vi "Apply Theme.vi"(8 "Error In":errorcluster, 10 "Override Root With (Empty)":string, 11 "Appearance Actor in":refnum<class "Appearance Actor.lvclass">) -> (0 "Error Out":errorcluster, 3 "Appearance Actor out":refnum<class "Appearance Actor.lvclass">)   [LabVIEW 2021, in "Appearance Actor.lvlib" / "Appearance Actor.lvclass"]
doc: "Apply the loaded theme to the current Actor.\n\nBy default, needs UI Control References to be listed in <B>Appearance Actor</B> internal data. But you can override this vi to do it your own way."
uses:
  Appearance Actor.lvclass
  Appearance Actor.lvclass/Appearance Actor.ctl
  Theme Classes/Generic Theme/Generic Theme.lvclass
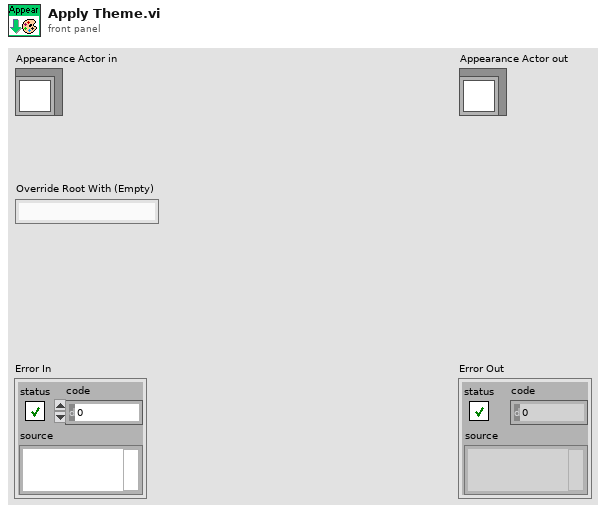
[diagram p1: front panel]
types:
  T1 = typedef "Appearance Actor.lvlib/Appearance Actor.lvclass/UI Controls--map.ctl" = map{string, T2}
  T2 = typedef "Appearance Actor.lvlib/Appearance Actor.lvclass/Element Controls--map.ctl" = map{string, T3}
  T3 = typedef "Appearance Actor.lvlib/Appearance Actor.lvclass/Controls--map.ctl" = map{string, refnum<vi>}
  T4 = typedef "Appearance Actor.lvlib/Appearance Actor.lvclass/UI Panes--map.ctl" = map{string, T5}
  T5 = typedef "Appearance Actor.lvlib/Appearance Actor.lvclass/Element Panes--map.ctl" = map{string, T6}
  T6 = typedef "Appearance Actor.lvlib/Appearance Actor.lvclass/Panes--map.ctl" = map{string, refnum<vi>}
  T7 = typedef "Appearance Actor.lvlib/Appearance Actor.lvclass/UI Splitters--map.ctl" = map{string, T8}
  T8 = typedef "Appearance Actor.lvlib/Appearance Actor.lvclass/Element Splitters--map.ctl" = map{string, T9}
  T9 = typedef "Appearance Actor.lvlib/Appearance Actor.lvclass/Splitters--map.ctl" = map{string, refnum<vi>}
  T10 = typedef "Appearance Actor.lvlib/Generic Theme.lvclass/Window Element--enum.ctl" = enum16{"None", "TB", "SM", "BP", "SB"}
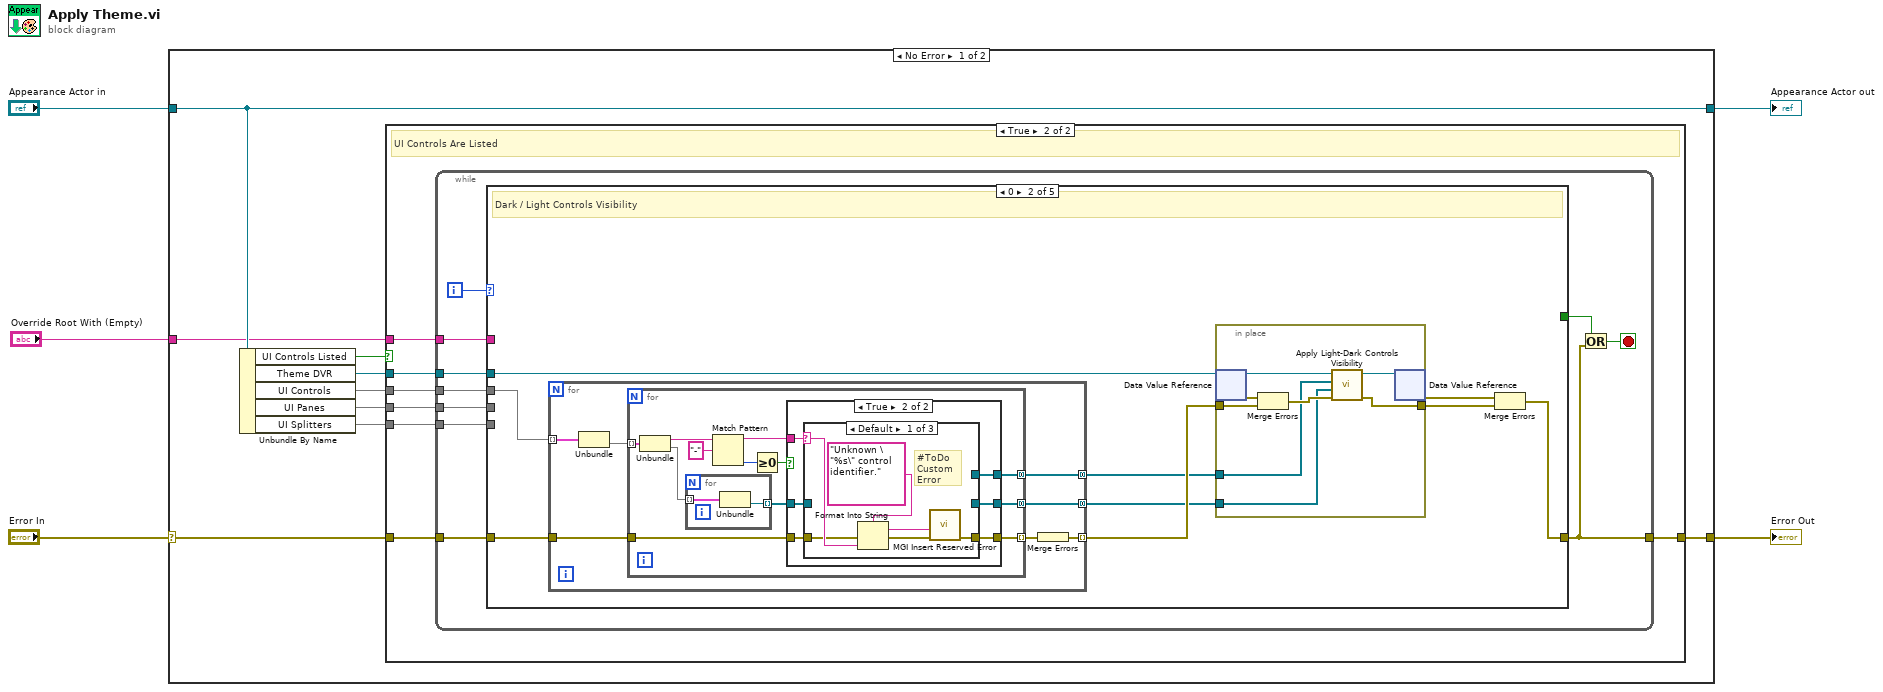
[diagram p0: block diagram]
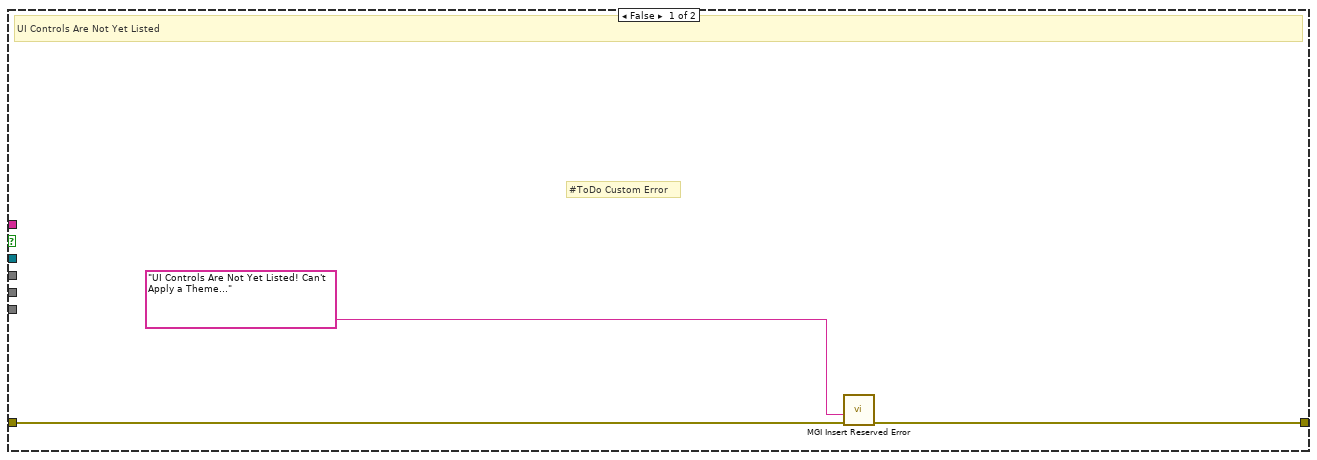
[diagram p2: hidden frame]
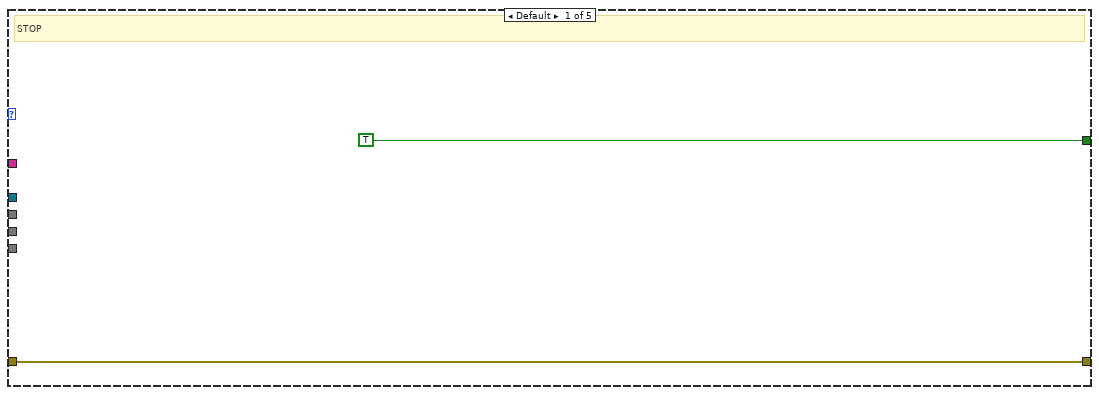
[diagram p3: hidden frame]
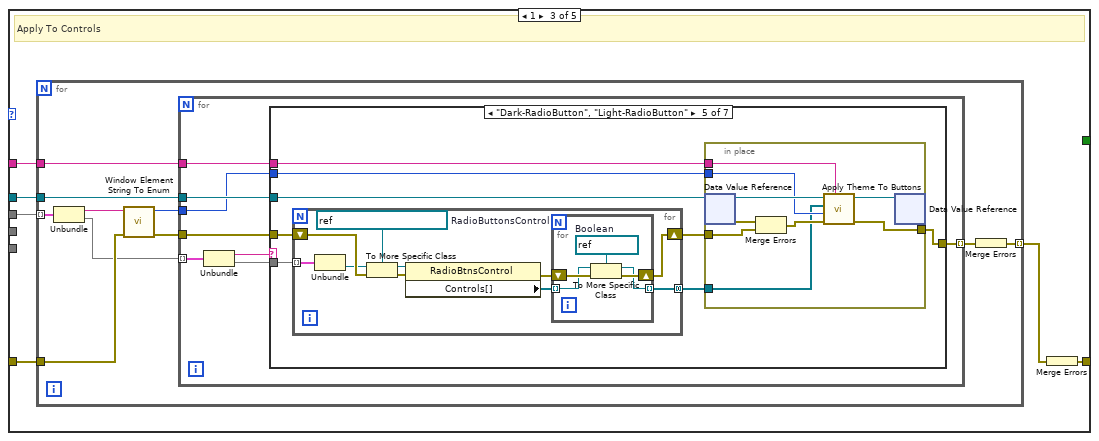
[diagram p7: hidden frame]
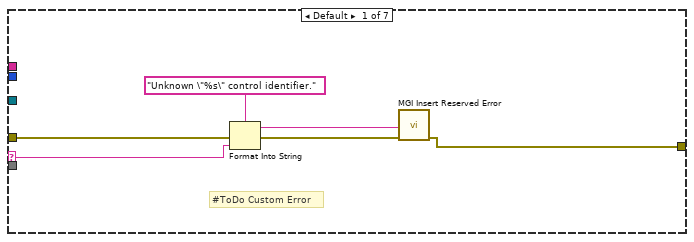
[diagram p8: hidden frame]
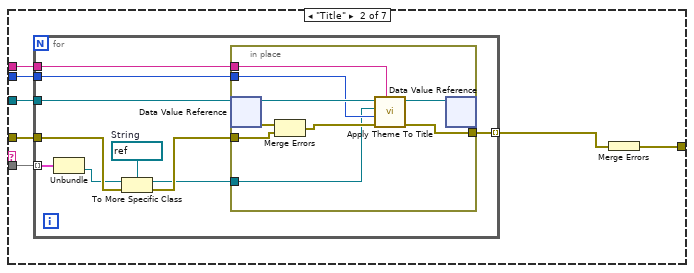
[diagram p9: hidden frame]
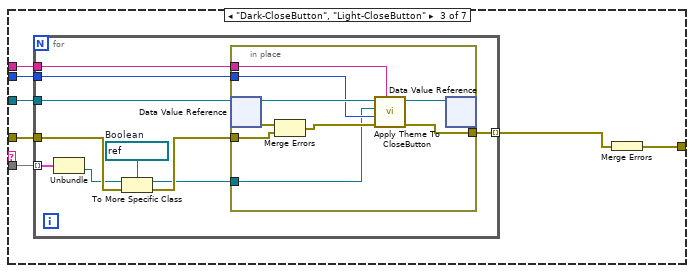
[diagram p10: hidden frame]
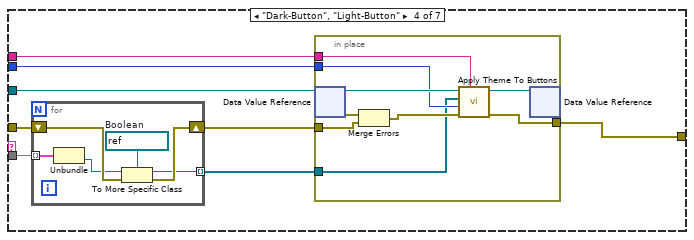
[diagram p11: hidden frame]
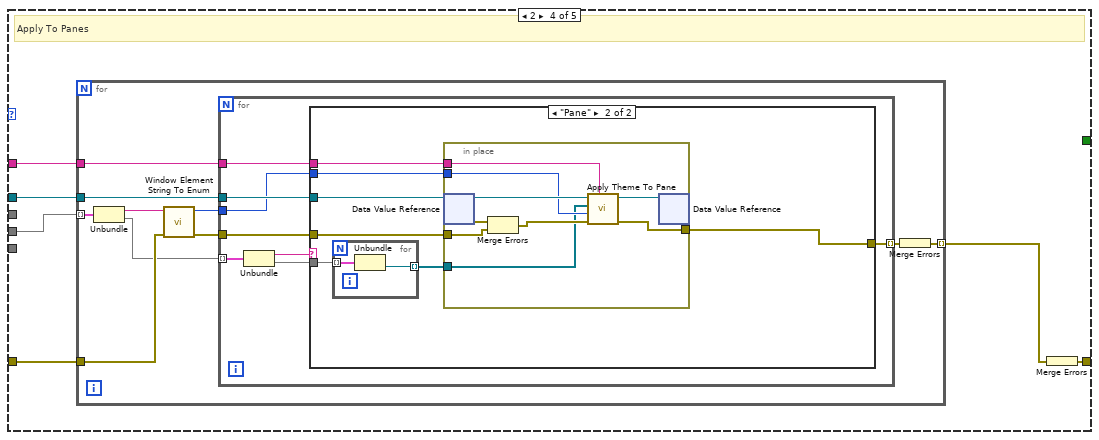
[diagram p14: hidden frame]
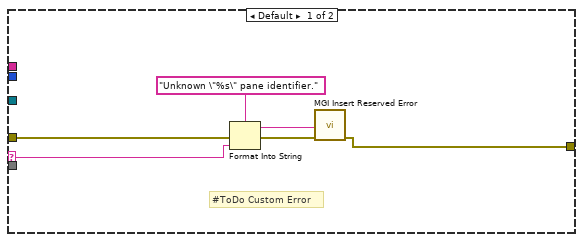
[diagram p15: hidden frame]
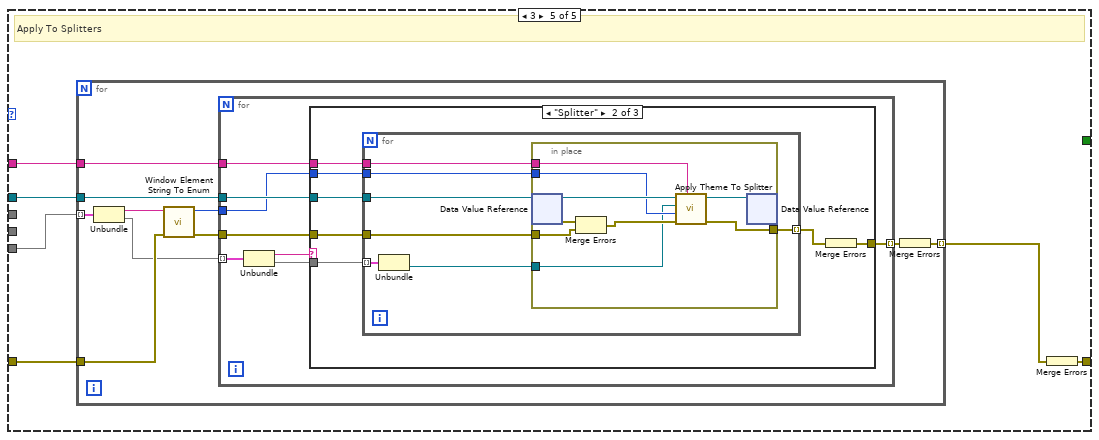
[diagram p16: hidden frame]
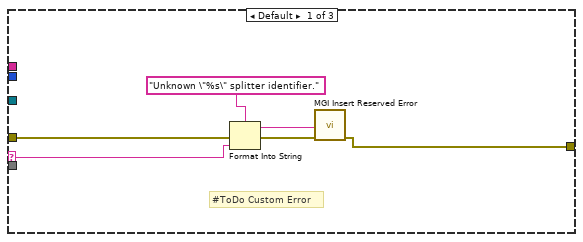
[diagram p17: hidden frame]
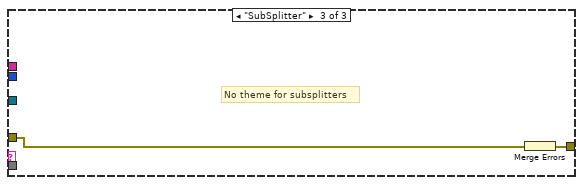
[diagram p18: hidden frame]
diagram:
  n1 = case shown="No Error" "Error In" {
    selector: "Error In" -> [w12 w335]
    tunnel: [w11 w335] -> w4
    tunnel: [w14 w334] -> w2
    tunnel: "Appearance Actor in" -> [w14 w334]
    tunnel: "Override Root With (Empty)" -> [w9 _]
    frame No Error {
      n2 = Unbundle By Name(w14) -> ("UI Controls Listed"=w10:bool, "Theme DVR"=w13:refnum<data-value>, "UI Controls"=w8:T1, "UI Panes"=w7:T4, "UI Splitters"=w6:T7)
      n3 = case shown="True" w10 {
        tunnel: w13 -> [_ w23]
        tunnel: w12 -> [w17 w21]
        tunnel: [w16 w24] -> w11
        tunnel: w9 -> [_ w22]
        tunnel: w8 -> [_ w20]
        tunnel: w7 -> [_ w19]
        tunnel: w6 -> [_ w18]
        frame False {
          # "#ToDo Custom Error"
          # "UI Controls Are Not Yet Listed"
          n4 = call <userlib>:"MGI Insert Reserved Error.vi"("Error In"=w17, "Error Description"="UI Controls Are Not Yet Listed! Can't Apply a Theme..." ("format string")) -> ("Error Out"=w16:errorcluster)  [unwired: 9 in]
        }
        frame True {
          # "UI Controls Are Listed"
          n5 = while {
            tunnel: w23 -> [w33]
            tunnel: w21 -> [w29]
            tunnel: [w30] -> w24
            tunnel: w22 -> [w28]
            tunnel: w20 -> [w27]
            tunnel: w19 -> [w26]
            tunnel: w18 -> [w25]
            i -> [w34]
            stop <- w31 stop-if-true
            n6 = case shown="0" w34 {
              tunnel: w33 -> [_ w42 w97 w236 w284]
              tunnel: [TRUE _ _ _ _] -> w32
              tunnel: w29 -> [w35 w40 w94 w234 w282]
              tunnel: [w35 w43 w92 w232 w280] -> w30
              tunnel: w28 -> [_ _ w95 w235 w283]
              tunnel: w27 -> [_ w41 w96 _ _]
              tunnel: w26 -> [_ _ _ w231 _]
              tunnel: w25 -> [_ _ _ _ w279]
              frame Default {
                # "STOP"
              }
              frame 0 {
                # "Dark / Light Controls Visibility"
                n7 = for {
                  tunnel: w41 -> [w52] mode=indexing
                  tunnel: w40 -> [w50]
                  tunnel: [w48] -> w39 mode=indexing
                  tunnel: [w47] -> w38 mode=concatenating
                  tunnel: [w46] -> w37 mode=concatenating
                  n8 = Unbundle(w52) -> ("Element Controls"=w51:T2)  [unwired: 1 out]
                  n9 = for {
                    tunnel: w51 -> [w64] mode=indexing
                    tunnel: w50 -> [w60]
                    tunnel: [w57] -> w49 mode=indexing
                    tunnel: [w54] -> w47 mode=concatenating
                    tunnel: [w53] -> w46 mode=concatenating
                    n10 = Unbundle(w64) -> ("Key"=w63:string, "Controls"=w56:T3)
                    n11 = for {
                      tunnel: w56 -> [w66] mode=indexing
                      tunnel: [w65] -> w55 mode=indexing
                      n12 = Unbundle(w66) -> ("Ctl Refnum"=w65:refnum<vi>)  [unwired: 1 out]
                    }
                    n13 = Match Pattern(string=w63, regular expression="-") -> (before substring=w58:string, offset past match=w61:i32)  [unwired: 1 in, 2 out]
                    n14 = Greater Or Equal To 0?(x=w61) -> (x >= 0?=w59:bool)
                    n15 = case shown="True" w59 {
                      tunnel: w60 -> [w67 w73]
                      tunnel: w58 -> [_ w71]
                      tunnel: [w67 w72] -> w57
                      tunnel: w55 -> [_ w70]
                      tunnel: [_ w69] -> w54
                      tunnel: [_ w68] -> w53
                      frame False {
                      }
                      frame True {
                        n16 = case shown="Default" w71 {
                          selector: w71 -> [w76 _ _]
                          tunnel: [w79 w81 w82] -> w72
                          tunnel: w73 -> [w75 w81 w82]
                          tunnel: w70 -> [_ w80 w83]
                          tunnel: [_ _ w83] -> w69
                          tunnel: [_ w80 _] -> w68
                          frame Default {
                            # "#ToDo Custom Error"
                            n17 = Format Into String(format string="Unknown \"%s\" control identifier.", error in=w75, w76) -> (resulting string=w77:string, error out=w74:errorcluster)  [unwired: 1 in]
                            n18 = call <userlib>:"MGI Insert Reserved Error.vi"("Error In"=w74, "Error Description"=w77) -> ("Error Out"=w79:errorcluster)  [unwired: 9 in]
                          }
                          frame "Light" {
                          }
                          frame "Dark" {
                          }
                        }
                      }
                    }
                  }
                  n19 = Merge Errors(w49) -> (w48:errorcluster)
                }
                n20 = in-place {
                  in-place-border: [w90] -> w44
                  in-place-border: w39 -> [w86]
                  in-place-border: w38 -> [w85]
                  in-place-border: w37 -> [w84]
                  n21 = in-place-dvr #1(w42) -> (w89:refnum<class "Generic Theme.lvclass">, w88:errorcluster)
                  n22 = Merge Errors(w88, w86) -> (w87:errorcluster)
                  n23 = call-dynamic "Apply Light-Dark Controls Visibility.vi"("Error In"=w87, "Dark Controls"=w85, "Light Controls"=w84, "Generic Theme in"=w89) -> ("Error Out"=w90:errorcluster, "Generic Theme out"=w91:refnum<class "Generic Theme.lvclass">)  [unwired: 6 in]
                  n24 = in-place-dvr #1(w91) -> (w45:errorcluster)  [unwired: 1 out]
                }
                n25 = Merge Errors(w45, w44) -> (w43:errorcluster)
              }
              frame 1 {
                # "Apply To Controls"
                n26 = for {
                  tunnel: w97 -> [w106]
                  tunnel: w96 -> [w105] mode=indexing
                  tunnel: w95 -> [w103]
                  tunnel: w94 -> [w107]
                  tunnel: [w98] -> w93 mode=indexing
                  n27 = Unbundle(w105) -> ("Key"=w102:string, "Element Controls"=w104:T2)
                  n28 = call "Window Element String To Enum.vi"("Error In"=w107, "Window Element Str"=w102) -> ("Error Out"=w100:errorcluster, "Window Element"=w101:T10)  [unwired: 8 in]
                  n29 = for {
                    tunnel: w106 -> [w115]
                    tunnel: w104 -> [w114] mode=indexing
                    tunnel: w103 -> [w113]
                    tunnel: w101 -> [w112]
                    tunnel: w100 -> [w111]
                    tunnel: [w108] -> w99 mode=indexing
                    n30 = Unbundle(w114) -> ("Key"=w110:string, "Controls"=w109:T3)
                    n31 = case shown="\"Dark-RadioButton\", \"Light-RadioButton\"" w110 {
                      selector: w110 -> [w118 _ _ _ _ _ _]
                      tunnel: w115 -> [_ w128 w154 w181 w204 _ _]
                      tunnel: w113 -> [_ w127 w153 w180 w203 _ _]
                      tunnel: w112 -> [_ w126 w152 w179 w202 _ _]
                      tunnel: w111 -> [w121 w125 w151 w178 w201 w229 w230]
                      tunnel: w109 -> [_ w124 w150 w177 w200 _ _]
                      tunnel: [w116 w122 w148 w174 w197 w229 w230] -> w108
                      frame Default {
                        # "#ToDo Custom Error"
                        n32 = Format Into String(format string="Unknown \"%s\" control identifier.", error in=w121, w118) -> (resulting string=w119:string, error out=w120:errorcluster)  [unwired: 1 in]
                        n33 = call <userlib>:"MGI Insert Reserved Error.vi"("Error In"=w120, "Error Description"=w119) -> ("Error Out"=w116:errorcluster)  [unwired: 9 in]
                      }
                      frame "Title" {
                        n34 = for {
                          tunnel: w128 -> [w138]
                          tunnel: w127 -> [w137]
                          tunnel: w126 -> [w136]
                          tunnel: w125 -> [w135]
                          tunnel: w124 -> [w131] mode=indexing
                          tunnel: [w129] -> w123 mode=indexing
                          w133 = refnum<vi> refnum  # String
                          n35 = Unbundle(w131) -> ("Ctl Refnum"=w130:refnum<vi>)  [unwired: 1 out]
                          n36 = To More Specific Class(target class=w133, reference=w130, error in=w135) -> (specific class reference=w132:refnum<vi>, error out=w134:errorcluster)
                          n37 = in-place {
                            in-place-border: [w144] -> w129
                            in-place-border: w137 -> [w143]
                            in-place-border: w136 -> [w142]
                            in-place-border: w134 -> [w140]
                            in-place-border: w132 -> [w139]
                            n38 = in-place-dvr #2(w138) -> (w147:refnum<class "Generic Theme.lvclass">, w146:errorcluster)
                            n39 = Merge Errors(w146, w140) -> (w141:errorcluster)
                            n40 = call-dynamic "Apply Theme To Title.vi"("Override Root With (Empty)"=w143, "Error In"=w141, "Window Element"=w142, "Title Ref"=w139, "Generic Theme in"=w147) -> ("Error Out"=w144:errorcluster, "Generic Theme out"=w145:refnum<class "Generic Theme.lvclass">)  [unwired: 5 in]
                            n41 = in-place-dvr #2(w145) -> ()  [unwired: 2 out]
                          }
                        }
                        n42 = Merge Errors(w123) -> (w122:errorcluster)
                      }
                      frame "Dark-CloseButton", "Light-CloseButton" {
                        n43 = for {
                          tunnel: w154 -> [w164]
                          tunnel: w153 -> [w163]
                          tunnel: w152 -> [w162]
                          tunnel: w151 -> [w161]
                          tunnel: w150 -> [w157] mode=indexing
                          tunnel: [w155] -> w149 mode=indexing
                          w159 = refnum<vi> refnum  # Boolean
                          n44 = Unbundle(w157) -> ("Ctl Refnum"=w156:refnum<vi>)  [unwired: 1 out]
                          n45 = To More Specific Class(target class=w159, reference=w156, error in=w161) -> (specific class reference=w158:refnum<vi>, error out=w160:errorcluster)
                          n46 = in-place {
                            in-place-border: [w170] -> w155
                            in-place-border: w163 -> [w169]
                            in-place-border: w162 -> [w168]
                            in-place-border: w160 -> [w166]
                            in-place-border: w158 -> [w165]
                            n47 = in-place-dvr #3(w164) -> (w173:refnum<class "Generic Theme.lvclass">, w172:errorcluster)
                            n48 = Merge Errors(w172, w166) -> (w167:errorcluster)
                            n49 = call-dynamic "Apply Theme To CloseButton.vi"("Override Root With (Empty)"=w169, "Error In"=w167, "Window Element"=w168, "CloseButton Ref"=w165, "Generic Theme in"=w173) -> ("Error Out"=w170:errorcluster, "Generic Theme out"=w171:refnum<class "Generic Theme.lvclass">)  [unwired: 5 in]
                            n50 = in-place-dvr #3(w171) -> ()  [unwired: 2 out]
                          }
                        }
                        n51 = Merge Errors(w149) -> (w148:errorcluster)
                      }
                      frame "Dark-Button", "Light-Button" {
                        n52 = for {
                          tunnel: w177 -> [w186] mode=indexing
                          tunnel: [w183] -> w175 mode=indexing
                          shift-right: [w185] -> w176
                          shift-left: w178 -> [w187]
                          w184 = refnum<vi> refnum  # Boolean
                          n53 = Unbundle(w186) -> ("Ctl Refnum"=w182:refnum<vi>)  [unwired: 1 out]
                          n54 = To More Specific Class(target class=w184, reference=w182, error in=w187) -> (specific class reference=w183:refnum<vi>, error out=w185:errorcluster)
                        }
                        n55 = in-place {
                          in-place-border: [w193] -> w174
                          in-place-border: w180 -> [w192]
                          in-place-border: w179 -> [w191]
                          in-place-border: w176 -> [w189]
                          in-place-border: w175 -> [w188]
                          n56 = in-place-dvr #4(w181) -> (w196:refnum<class "Generic Theme.lvclass">, w195:errorcluster)
                          n57 = Merge Errors(w195, w189) -> (w190:errorcluster)
                          n58 = call-dynamic "Apply Theme To Buttons.vi"("Override Root With (Empty)"=w192, "Error In"=w190, "Window Element"=w191, "Buttons Ref"=w188, "Generic Theme in"=w196) -> ("Error Out"=w193:errorcluster, "Generic Theme out"=w194:refnum<class "Generic Theme.lvclass">)  [unwired: 5 in]
                          n59 = in-place-dvr #4(w194) -> ()  [unwired: 2 out]
                        }
                      }
                      frame "Dark-RadioButton", "Light-RadioButton" {
                        n60 = for {
                          tunnel: w200 -> [w213] mode=indexing
                          tunnel: [w205] -> w198 mode=concatenating
                          shift-right: [w206] -> w199
                          shift-left: w201 -> [w214]
                          w212 = refnum<vi> refnum  # RadioButtonsControl
                          n61 = Unbundle(w213) -> ("Ctl Refnum"=w211:refnum<vi>)  [unwired: 1 out]
                          n62 = To More Specific Class(target class=w212, reference=w211, error in=w214) -> (specific class reference=w210:refnum<vi>, error out=w209:errorcluster)
                          n63 = property class="RadioBtnsControl"(reference=w210, error in=w209) -> (error out=w207:errorcluster, "Controls[]"=w208:refnum<vi>[])  [unwired: 1 out]
                          n64 = for {
                            tunnel: w208 -> [w217] mode=indexing
                            shift-right: [w218] -> w206
                            shift-left: w207 -> [w219]
                            tunnel: [w216] -> w205 mode=indexing
                            w215 = refnum<vi> refnum  # Boolean
                            n65 = To More Specific Class(target class=w215, reference=w217, error in=w219) -> (specific class reference=w216:refnum<vi>, error out=w218:errorcluster)
                          }
                        }
                        n66 = in-place {
                          in-place-border: [w225] -> w197
                          in-place-border: w203 -> [w224]
                          in-place-border: w202 -> [w223]
                          in-place-border: w199 -> [w221]
                          in-place-border: w198 -> [w220]
                          n67 = in-place-dvr #5(w204) -> (w228:refnum<class "Generic Theme.lvclass">, w227:errorcluster)
                          n68 = Merge Errors(w227, w221) -> (w222:errorcluster)
                          n69 = call-dynamic "Apply Theme To Buttons.vi"("Override Root With (Empty)"=w224, "Error In"=w222, "Window Element"=w223, "Buttons Ref"=w220, "Generic Theme in"=w228) -> ("Error Out"=w225:errorcluster, "Generic Theme out"=w226:refnum<class "Generic Theme.lvclass">)  [unwired: 5 in]
                          n70 = in-place-dvr #5(w226) -> ()  [unwired: 2 out]
                        }
                      }
                      frame "SubPanel" {
                        # "No theme for SubPanels"
                      }
                      frame "Icon" {
                        # "No theme for Icon"
                      }
                    }
                  }
                  n71 = Merge Errors(w99) -> (w98:errorcluster)
                }
                n72 = Merge Errors(w93) -> (w92:errorcluster)
              }
              frame 2 {
                # "Apply To Panes"
                n73 = for {
                  tunnel: w236 -> [w245]
                  tunnel: w231 -> [w244] mode=indexing
                  tunnel: w235 -> [w242]
                  tunnel: w234 -> [w246]
                  tunnel: [w237] -> w233 mode=indexing
                  n74 = Unbundle(w244) -> ("Key"=w241:string, "Element Panes"=w243:T5)
                  n75 = call "Window Element String To Enum.vi"("Error In"=w246, "Window Element Str"=w241) -> ("Error Out"=w239:errorcluster, "Window Element"=w240:T10)  [unwired: 8 in]
                  n76 = for {
                    tunnel: w245 -> [w254]
                    tunnel: w243 -> [w253] mode=indexing
                    tunnel: w242 -> [w252]
                    tunnel: w240 -> [w251]
                    tunnel: w239 -> [w250]
                    tunnel: [w247] -> w238 mode=indexing
                    n77 = Unbundle(w253) -> ("Key"=w249:string, "Panes"=w248:T6)
                    n78 = case shown="\"Pane\"" w249 {
                      selector: w249 -> [w257 _]
                      tunnel: w254 -> [_ w267]
                      tunnel: w252 -> [_ w266]
                      tunnel: w251 -> [_ w265]
                      tunnel: w250 -> [w260 w261]
                      tunnel: w248 -> [_ w264]
                      tunnel: [w255 w262] -> w247
                      frame Default {
                        # "#ToDo Custom Error"
                        n79 = Format Into String(format string="Unknown \"%s\" pane identifier.", error in=w260, w257) -> (resulting string=w258:string, error out=w259:errorcluster)  [unwired: 1 in]
                        n80 = call <userlib>:"MGI Insert Reserved Error.vi"("Error In"=w259, "Error Description"=w258) -> ("Error Out"=w255:errorcluster)  [unwired: 9 in]
                      }
                      frame "Pane" {
                        n81 = for {
                          tunnel: w264 -> [w269] mode=indexing
                          tunnel: [w268] -> w263 mode=indexing
                          n82 = Unbundle(w269) -> ("Pane Refnum"=w268:refnum<vi>)  [unwired: 1 out]
                        }
                        n83 = in-place {
                          in-place-border: [w275] -> w262
                          in-place-border: w266 -> [w274]
                          in-place-border: w265 -> [w273]
                          in-place-border: w261 -> [w271]
                          in-place-border: w263 -> [w270]
                          n84 = in-place-dvr #6(w267) -> (w278:refnum<class "Generic Theme.lvclass">, w277:errorcluster)
                          n85 = Merge Errors(w277, w271) -> (w272:errorcluster)
                          n86 = call-dynamic "Apply Theme To Pane.vi"("Override Root With (Empty)"=w274, "Error In"=w272, "Window Element"=w273, "Pane Refs"=w270, "Generic Theme in"=w278) -> ("Error Out"=w275:errorcluster, "Generic Theme out"=w276:refnum<class "Generic Theme.lvclass">)  [unwired: 5 in]
                          n87 = in-place-dvr #6(w276) -> ()  [unwired: 2 out]
                        }
                      }
                    }
                  }
                  n88 = Merge Errors(w238) -> (w237:errorcluster)
                }
                n89 = Merge Errors(w233) -> (w232:errorcluster)
              }
              frame 3 {
                # "Apply To Splitters"
                n90 = for {
                  tunnel: w284 -> [w293]
                  tunnel: w279 -> [w292] mode=indexing
                  tunnel: w283 -> [w290]
                  tunnel: w282 -> [w294]
                  tunnel: [w285] -> w281 mode=indexing
                  n91 = Unbundle(w292) -> ("Key"=w289:string, "Element Splitters"=w291:T8)
                  n92 = call "Window Element String To Enum.vi"("Error In"=w294, "Window Element Str"=w289) -> ("Error Out"=w287:errorcluster, "Window Element"=w288:T10)  [unwired: 8 in]
                  n93 = for {
                    tunnel: w293 -> [w302]
                    tunnel: w291 -> [w301] mode=indexing
                    tunnel: w290 -> [w300]
                    tunnel: w288 -> [w299]
                    tunnel: w287 -> [w298]
                    tunnel: [w295] -> w286 mode=indexing
                    n94 = Unbundle(w301) -> ("Key"=w297:string, "Splitters"=w296:T9)
                    n95 = case shown="\"Splitter\"" w297 {
                      selector: w297 -> [w305 _ _]
                      tunnel: w302 -> [_ w315 _]
                      tunnel: w300 -> [_ w314 _]
                      tunnel: w299 -> [_ w313 _]
                      tunnel: w298 -> [w308 w312 w332]
                      tunnel: w296 -> [_ w311 _]
                      tunnel: [w303 w309 w333] -> w295
                      frame Default {
                        # "#ToDo Custom Error"
                        n96 = Format Into String(format string="Unknown \"%s\" splitter identifier.", error in=w308, w305) -> (resulting string=w306:string, error out=w307:errorcluster)  [unwired: 1 in]
                        n97 = call <userlib>:"MGI Insert Reserved Error.vi"("Error In"=w307, "Error Description"=w306) -> ("Error Out"=w303:errorcluster)  [unwired: 9 in]
                      }
                      frame "Splitter" {
                        n98 = for {
                          tunnel: w315 -> [w322]
                          tunnel: w314 -> [w321]
                          tunnel: w313 -> [w320]
                          tunnel: w312 -> [w319]
                          tunnel: w311 -> [w318] mode=indexing
                          tunnel: [w316] -> w310 mode=indexing
                          n99 = Unbundle(w318) -> ("Splitter Refnum"=w317:refnum<vi>)  [unwired: 1 out]
                          n100 = in-place {
                            in-place-border: [w328] -> w316
                            in-place-border: w321 -> [w327]
                            in-place-border: w320 -> [w326]
                            in-place-border: w319 -> [w324]
                            in-place-border: w317 -> [w323]
                            n101 = in-place-dvr #7(w322) -> (w331:refnum<class "Generic Theme.lvclass">, w330:errorcluster)
                            n102 = Merge Errors(w330, w324) -> (w325:errorcluster)
                            n103 = call-dynamic "Apply Theme To Splitter.vi"("Override Root With (Empty)"=w327, "Error In"=w325, "Window Element"=w326, "Splitter Ref"=w323, "Generic Theme in"=w331) -> ("Error Out"=w328:errorcluster, "Generic Theme out"=w329:refnum<class "Generic Theme.lvclass">)  [unwired: 5 in]
                            n104 = in-place-dvr #7(w329) -> ()  [unwired: 2 out]
                          }
                        }
                        n105 = Merge Errors(w310) -> (w309:errorcluster)
                      }
                      frame "SubSplitter" {
                        # "No theme for subsplitters"
                        n106 = Merge Errors(w332) -> (w333:errorcluster)
                      }
                    }
                  }
                  n107 = Merge Errors(w286) -> (w285:errorcluster)
                }
                n108 = Merge Errors(w281) -> (w280:errorcluster)
              }
            }
            n109 = Or(x=w32, y=w30) -> (x .or. y?=w31:bool)
          }
        }
      }
    }
    frame Error {
    }
  }
  "Error Out" <- w4
  "Appearance Actor out" <- w2
